vi "Validate Virt Instrs CFG.vi"(8 "error in":errorcluster, 11 "<JSON>":string) -> (0 "error out":errorcluster, 2 "Is Valid?":bool)   [LabVIEW 2023, in "Configuration UI Actor.lvlib" / "Configuration UI Actor.lvclass"]
uses:
  Configuration UI Actor.lvclass
  HAL GOOP4/Virtual Instrument Base/Virt Instr Base.lvclass
  86413ab1-e05c-4a15-b757-f1181f9f1753.vi
  <vilib>/JDP Science/JSONtext/Find Item.vi
  <vilib>/JDP Science/JSONtext/Next JSON Value.vi
  <vilib>/JDP Science/JSONtext/String Subset.vi
  <vilib>/JDP Science/JSONtext/Parsing/Advance past next JSON Value (inlined COPY).vi
  <vilib>/JDP Science/JSONtext/Parsing/Advance past whitespace.vi
  <vilib>/JDP Science/JSONtext/Parsing/Advance past String.vi
  <vilib>/JDP Science/JSONtext/Parsing/Advance past Number.vi
  <vilib>/JDP Science/JSONtext/Parsing/Advance past Line Ending.vi
  <vilib>/JDP Science/JSONtext/Parsing/Parse Full Path or Item Name.vi
  <vilib>/JDP Science/JSONtext/Parsing/Advance past Array.vi
  <vilib>/JDP Science/JSONtext/Parsing/Advance past Object.vi
  <vilib>/JDP Science/JSONtext/support/Error Cluster From Code.vi
  <vilib>/JDP Science/JSONtext/Offset/Find Item Locations by Path.vi
  <vilib>/JDP Science/JSONtext/JSON text to Variant.vi
  <vilib>/Utility/error.llb/Error Cluster From Error Code.vi
  <vilib>/JDP Science/JSONtext/LVClass Serializer/JSONtext LVClass Serializer.lvclass
  <vilib>/ErrorRing/Error Ring.xnode
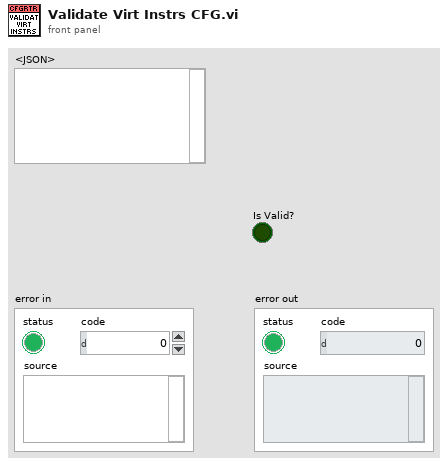
[diagram p1: front panel]
types:
  T1 = cluster{"Target Ident":string, "Instr Ident":string, "Const Action Data":string, "Class":string}[]
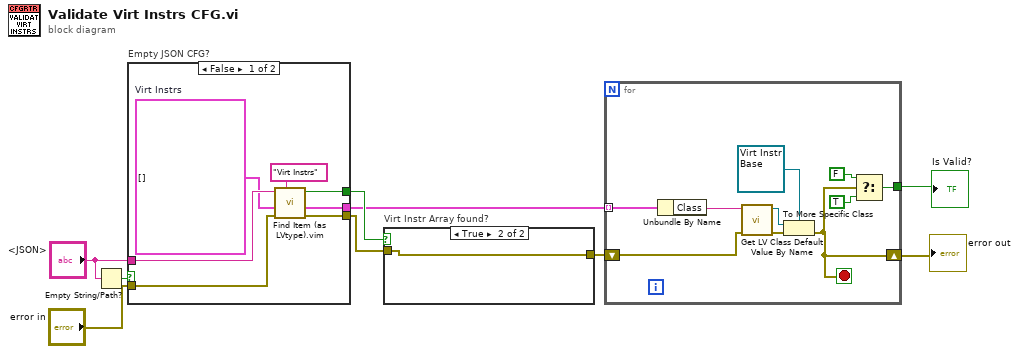
[diagram p0: block diagram]
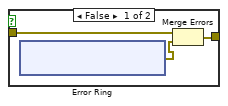
[diagram p2: hidden frame]
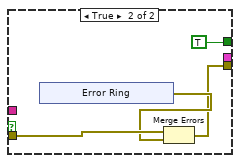
[diagram p3: hidden frame]
diagram:
  n1 = Empty String/Path?(string/path="<JSON>") -> (empty?=w9:bool)
  n2 = case "Empty JSON CFG?" shown="False" w9 {
    tunnel: "error in" -> [w16 w20]
    tunnel: [w14 w18] -> w5
    tunnel: "<JSON>" -> [w15 _]
    tunnel: [w11 _] -> w4
    tunnel: [w10 TRUE ("Found")] -> w6
    frame False {
      w13 = T1 []  # Virt Instrs
      n3 = call "Find Item (as LVtype).vim"("$Path or Item Name"="Virt Instrs", "error in (no error)"=w16, "Data Type and Default Value"=w13, "JSON"=w15) -> ("error out"=w14:errorcluster, "Data"=w11:T1, "Found"=w10:bool)  [unwired: 4 in, 1 out]
    }
    frame True {
      n4 = xnode "Error Ring"() -> ("error out"=w19:errorcluster)
      n5 = Merge Errors(w20, w19) -> (w18:errorcluster)
    }
  }
  n6 = case "Virt Instr Array found?" shown="True" w6 {
    tunnel: [w28 w34] -> w3
    tunnel: w5 -> [w26 w34]
    frame False {
      n7 = xnode "Error Ring"() -> ("error out"=w27:errorcluster)
      n8 = Merge Errors(w26, w27) -> (w28:errorcluster)
    }
    frame True {
    }
  }
  n9 = for {
    tunnel: w4 -> [w41] mode=indexing
    shift-right: [w38] -> w2
    shift-left: w3 -> [w39]
    tunnel: [w35] -> w1
    stop <- w38 stop-if-true
    n10 = Unbundle By Name(w41) -> ("Class"=w40:string)
    n11 = call <vilib>:"Get LV Class Default Value By Name.vi"("error in (no error)"=w39, "class name"=w40) -> ("error out"=w44:errorcluster, "object"=w42:refnum<class>)  [unwired: 8 in]
    n12 = To More Specific Class(target class=refnum<class "Virt Instr Base.lvclass"> refnum ("HAL GOOP4.lvlib:Virtual Instrument Base.lvclass"), reference=w42, error in=w44) -> (error out=w38:errorcluster)  [unwired: 1 out]
    n13 = Select(t=FALSE, s=w38, f=TRUE) -> (s? t:f=w35:bool)
  }
  "error out" <- w2
  "Is Valid?" <- w1
